vi "NestedFact1.vi"() -> ()   [LabVIEW 2019, in "TestSuiteTest.lvlib" / "Support.lvlib" / "FakeLibrary.lvlib" / "NestedLibrary.lvlib"]
uses:
  NestedLibrary.lvlib
panel:
  out "error out":errorcluster
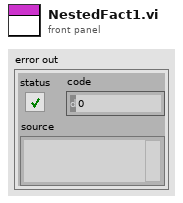
[diagram p1: front panel]
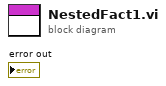
[diagram p0: block diagram]
diagram:
